vi "Get Identifier.vi"(8 "error in (no error)":errorcluster, 11 "Execution Unit Implementation in":refnum<class "Execution Unit.lvclass">) -> (0 "error out":errorcluster, 2 "Identifier":string, 3 "Execution Unit Implementation out":refnum<class "Execution Unit.lvclass">)   [LabVIEW 2020, in "Ballard MIL-STD-1553 Engine.lvlib" / "Implementation.lvlib" / "Execution Unit.lvclass"]
uses:
  Execution Unit.lvclass
  Execution Unit.lvclass/Execution Unit.ctl
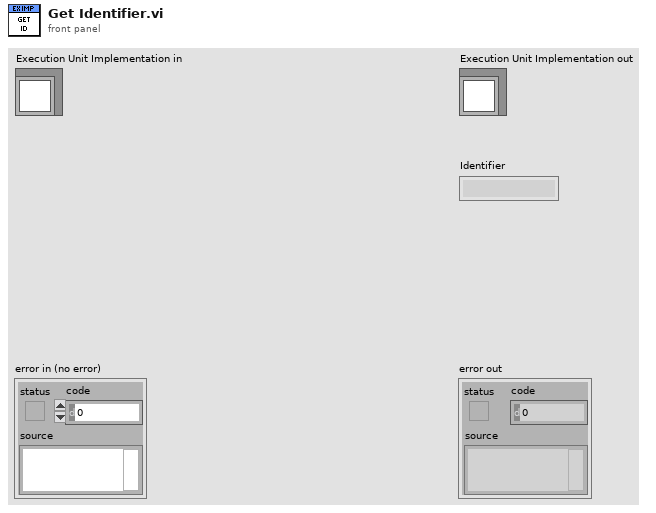
[diagram p1: front panel]
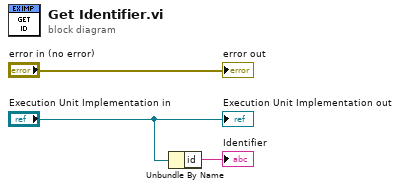
[diagram p0: block diagram]
diagram:
  n1 = Unbundle By Name("Execution Unit Implementation in") -> ("id"=→"Identifier":string)
  "error out" <- "error in (no error)"
  "Execution Unit Implementation out" <- "Execution Unit Implementation in"
